vi "RSZVB Get Automatic Generator Attenuator.vi"(8 "error in (no error)":errorcluster {"code" format="%.0x"}, 9 "Port (1)":i32=1, 10 "Channel (1)":i32=1, 11 "VISA session":refnum<visa-resource-name>) -> (0 "error out":errorcluster {"code" format="%.0x"}, 1 "Automatic Attenuation":bool, 3 "dup VISA session":refnum<visa-resource-name>)   [LabVIEW 2011]
doc: "This VI gets whether the attenuation factor for the generated wave at test port no. <Pt> is set manually or automatically. \n\nNote(s):\n\n(1) This VI can be used only with R&S ZVA and ZVB instruments.\n\nRemote-control command(s):\nSOURce<Ch>:POWer<Pt>:ATTenuation:AUTO?"
uses:
  _utility/RSZVB Global Data.vi
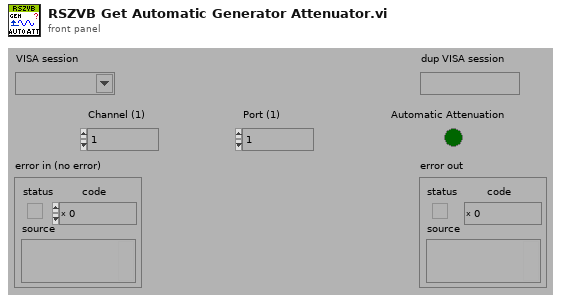
[diagram p1: front panel]
types:
  T1 = cluster{"Error Checking (T: On)":bool, "Installed Options":string[], "Data Valid?":bool, "Ports":i32, "Model":string[], "Option Checking (T: On)":bool}[]
  T2 = cluster{"Error Checking (T: On)":bool, "Installed Options":string[], "Data Valid?":bool, "Ports":i32, "Model":string[], "Option Checking (T: On)":bool}
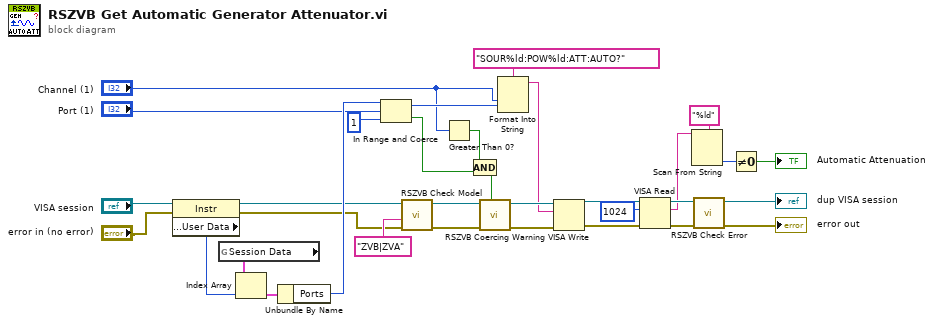
[diagram p0: block diagram]
diagram:
  n1 = property class="Instr"(reference="VISA session", error in="error in (no error)") -> (reference out=w20:refnum<visa-resource-name>, error out=w19:errorcluster, "General Settings:User Data"=w22:u32)
  n2 = global read "RSZVB Global Data.vi" "Session Data"() -> (w23:T1)
  n3 = Index Array(array=w23, index=w22) -> (element=w24:T2)
  n4 = Unbundle By Name(w24) -> ("Ports"=w21:i32)
  n5 = In Range and Coerce(upper limit=w21, x="Port (1)", lower limit=1) -> (coerced(x)=w17:i32, In Range?=w18:bool)
  n6 = call "RSZVB Check Model.vi"("error in (no error)"=w19, "Model"="ZVB|ZVA" ("Options"), "VISA session"=w20) -> ("error out"=w27:errorcluster, "dup VISA session"=w26:refnum<visa-resource-name>)  [unwired: 7 in]
  n7 = Greater Than 0?(x="Channel (1)") -> (x > 0?=w28:bool)
  n8 = Compound Arithmetic op=AND(w28, w18) -> (w30:bool)
  n9 = call "RSZVB Coercing Warning.vi"("In Range?"=w30, "error in (no error)"=w27, "VISA session"=w26) -> ("error out"=w31:errorcluster, "dup VISA session"=w32:refnum<visa-resource-name>)  [unwired: 7 in]
  n10 = Format Into String(format string="SOUR%ld:POW%ld:ATT:AUTO?", "Channel (1)", w17) -> (resulting string=w29:string)  [unwired: 2 in, 1 out]
  n11 = VISA Write(VISA resource name=w32, write buffer=w29, error in (no error)=w31) -> (VISA resource name out=w5:refnum<visa-resource-name>, error out=w4:errorcluster)  [unwired: 1 out]
  n12 = VISA Read(VISA resource name=w5, byte count=u32 1024 ("byte count (0)"), error in (no error)=w4) -> (VISA resource name out=w10:refnum<visa-resource-name>, read buffer=w7:string, error out=w9:errorcluster)  [unwired: 1 out]
  n13 = Scan From String(format string="%ld", input string=w7) -> (output 1=w6:i32)  [unwired: 3 in, 3 out]
  n14 = call "RSZVB Check Error.vi"("error in (no error)"=w9, "VISA session"=w10) -> ("error out"=→"error out":errorcluster, "dup VISA session"=→"dup VISA session":refnum<visa-resource-name>)  [unwired: 8 in]
  n15 = Not Equal To 0?(x=w6) -> (x != 0?=→"Automatic Attenuation":bool)
